vi "test Loopback.vi"(8 "error in (no error)":errorcluster, 11 "TestCase in":refnum<class "SLSC EDS System Tests.lvclass">) -> (0 "error out":errorcluster, 3 "TestCase out":refnum<class "SLSC EDS System Tests.lvclass">)   [LabVIEW 2015, in "SLSC EDS System Tests.lvclass"]
uses:
  SLSC EDS System Tests.lvclass
  niveristand-custom-device-testing-tools/Loopback/Loopback.lvclass
  <vilib>/addons/_JKI Toolkits/VI Tester/TestCase.llb/TestCase.lvclass
  niveristand-custom-device-testing-tools/VeriStandTestCase/VeriStandTestCase.lvclass
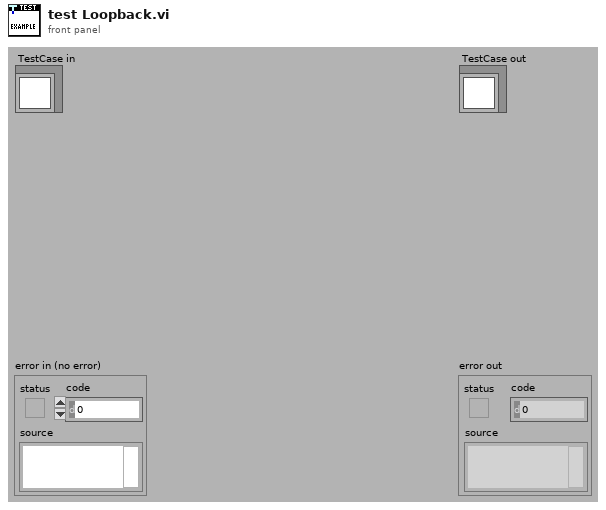
[diagram p1: front panel]
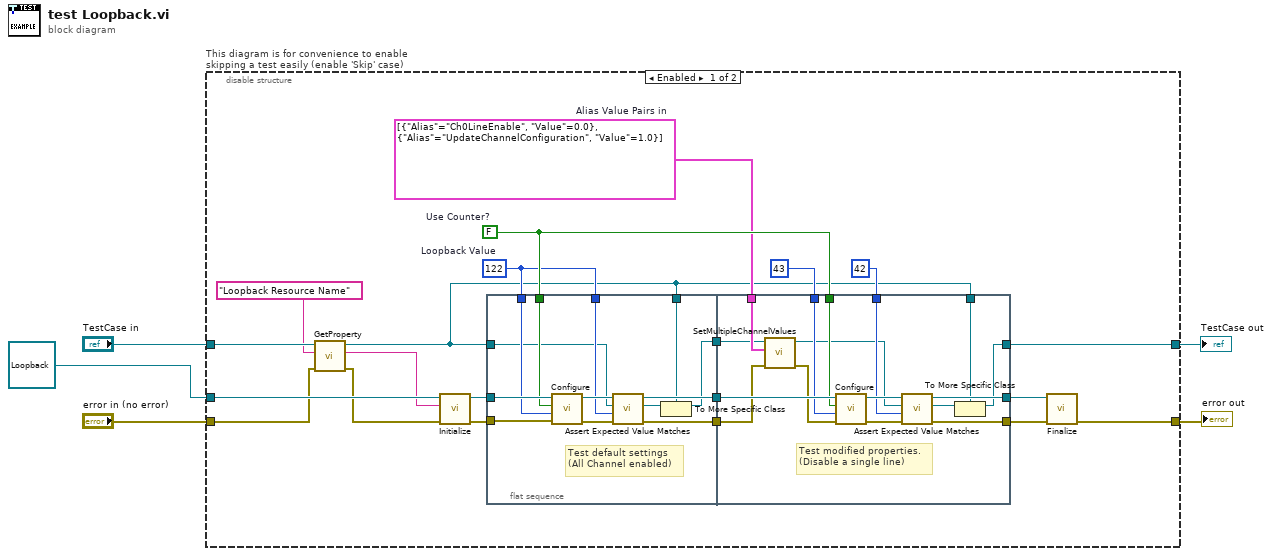
[diagram p0: block diagram]
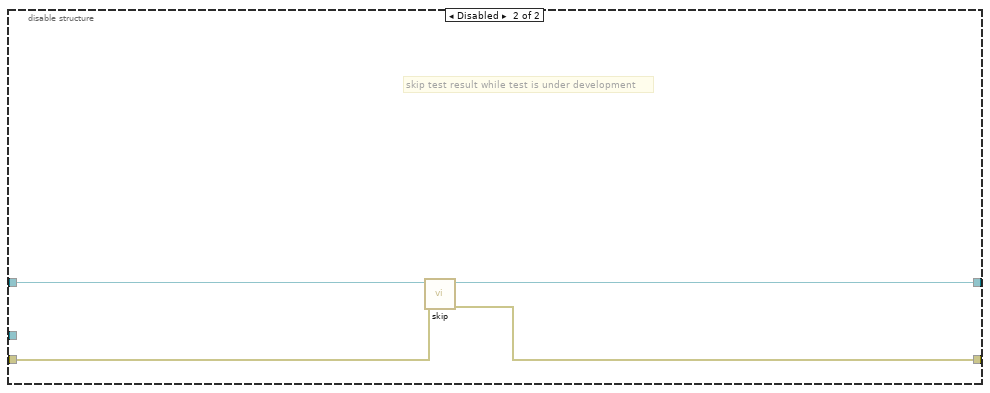
[diagram p2: hidden frame]
diagram:
  n1 = disable-structure "This diagram is for convenience to enable skipping a test easily (enable 'Skip' case)" shown="Enabled" {
    disable-tunnel: "TestCase in" -> [w11 w59]
    disable-tunnel: [w13 w57] -> w1
    disable-tunnel: [w15 w58] -> w4
    disable-tunnel: "error in (no error)" -> [w9 w56]
    disable-tunnel: refnum<class "Loopback.lvclass"> refnum ("Loopback.lvclass") -> [w21 _]
    frame Enabled {
      w25 = cluster{"Alias":string, "Value":dbl}[] [{"Alias"="Ch0LineEnable", "Value"=0.0}, {"Alias"="UpdateChannelConfiguration", "Value"=1.0}]  # Alias Value Pairs in
      w22 = u8 122  # Loopback Value
      w26 = FALSE  # Use Counter?
      n2 = call "GetProperty.vi"("error in (no error)"=w9, "key"="Loopback Resource Name", "VeriStandTestCase in"=w11) -> ("error out"=w8:errorcluster, "value"=w7:string, "VeriStandTestCase out"=w10:refnum<class "SLSC EDS System Tests.lvclass">)  [unwired: 6 in]
      n3 = call-dynamic "Initialize.vi"("error in (no error)"=w8, "Resource Name in"=w7, "Loopback in"=w21) -> ("error out"=w20:errorcluster, "Loopback out"=w19:refnum<class "Loopback.lvclass">)  [unwired: 7 in]
      n4 = flat-sequence {
        tunnel: w10 -> [w30]
        tunnel: w20 -> [w38]
        tunnel: w22 -> [w37]
        tunnel: w26 -> [w36]
        tunnel: w22 -> [w31]
        tunnel: w19 -> [w39]
        tunnel: [w33] -> w18
        tunnel: [w32] -> w17
        tunnel: [w28] -> w12
        tunnel: w10 -> [w27]
        tunnel: w26 -> [w52]
        tunnel: w25 -> [w47]
        tunnel: u8 43 ("Value") -> [w53]
        tunnel: u8 42 ("Expected Value") -> [w49]
        tunnel: w18 -> [w46]
        tunnel: w17 -> [w54]
        tunnel: [w51] -> w16
        tunnel: [w48] -> w14
        tunnel: [w42] -> w13
        tunnel: w12 -> [w43]
        tunnel: w10 -> [w40]
        frame #0 {
          # "Test default settings\n(All Channel enabled)"
          n5 = call-dynamic "Configure.vi"("error in (no error)"=w38, "Value in"=w37, "Use Counter?"=w36, "Loopback in"=w39) -> ("error out"=w34:errorcluster, "Loopback out"=w35:refnum<class "Loopback.lvclass">)  [unwired: 6 in]
          n6 = call-dynamic "Assert Expected Value Matches.vi"("error in (no error)"=w34, "Expected Value"=w31, "TestCase in"=w30, "Loopback in"=w35) -> ("error out"=w33:errorcluster, "TestCase out"=w29:refnum<class "TestCase.lvclass">, "Loopback out"=w32:refnum<class "Loopback.lvclass">)  [unwired: 5 in]
          n7 = To More Specific Class(target class=w27, reference=w29) -> (specific class reference=w28:refnum<class "SLSC EDS System Tests.lvclass">)  [unwired: 1 in, 1 out]
        }
        frame #1 {
          # "Test modified properties.\n(Disable a single line)"
          n8 = call-dynamic "SetMultipleChannelValues.vi"("error in (no error)"=w46, "Channel Key Value Pairs in"=w47, "VeriStandTestCase in"=w43) -> ("error out"=w45:errorcluster, "VeriStandTestCase out"=w44:refnum<class "SLSC EDS System Tests.lvclass">)  [unwired: 7 in]
          n9 = call-dynamic "Configure.vi"("error in (no error)"=w45, "Value in"=w53, "Use Counter?"=w52, "Loopback in"=w54) -> ("error out"=w55:errorcluster, "Loopback out"=w50:refnum<class "Loopback.lvclass">)  [unwired: 6 in]
          n10 = call-dynamic "Assert Expected Value Matches.vi"("error in (no error)"=w55, "Expected Value"=w49, "TestCase in"=w44, "Loopback in"=w50) -> ("error out"=w51:errorcluster, "TestCase out"=w41:refnum<class "TestCase.lvclass">, "Loopback out"=w48:refnum<class "Loopback.lvclass">)  [unwired: 5 in]
          n11 = To More Specific Class(target class=w40, reference=w41) -> (specific class reference=w42:refnum<class "SLSC EDS System Tests.lvclass">)  [unwired: 1 in, 1 out]
        }
      }
      n12 = call-dynamic "Finalize.vi"("error in (no error)"=w16, "Loopback in"=w14) -> ("error out"=w15:errorcluster)  [unwired: 8 in, 1 out]
    }
    frame Disabled {
      # "skip test result while test is under development"
      n13 = call <vilib>:"skip.vi"("error in (no error)"=w56, "TestCase in"=w59) -> ("error out"=w58:errorcluster, "TestCase out"=w57:refnum<class "SLSC EDS System Tests.lvclass">)  [unwired: 8 in]
    }
  }
  "error out" <- w4
  "TestCase out" <- w1
